vi "Simulador Circuito RLC-2.0.vi"() -> ()   [LabVIEW 2020]
uses:
  <vilib>/Utility/file.llb/Read Delimited Spreadsheet (DBL).vi
  <vilib>/measure/NI_MABase.lvlib
panel:
  in  "C":dbl
  in  "L":dbl
  in  "R":dbl
  in  "Gerar ondas\nde saída":bool
  out "Tensão no Capacitor":cluster{dbl[], "Y":dbl[]}[](graph)
  out "Corrente":cluster{dbl[], "Y":dbl[]}[](graph)
  in  "Arquivo texto da onda":path
  out "Onda de entrada":cluster{dbl[], "Y":dbl[]}(graph)
  in  "Duty Cicle":dbl
  in  "Informação da amostragem":T1={"Taxa de amostragem"=1000.0, "N° de amostras"=10000.0} {"N° de amostras" format="%#.6g"; "Taxa de amostragem" format="%#.6g"}
  in  "Gerar onda \nde Entrada":bool
  in  "Tipo de Onda":u16(ring) items=["Onda qualquer", "Senoidal", "Quadrada", ""]
  in  "Amplitude":dbl
  in  "Frequência":dbl
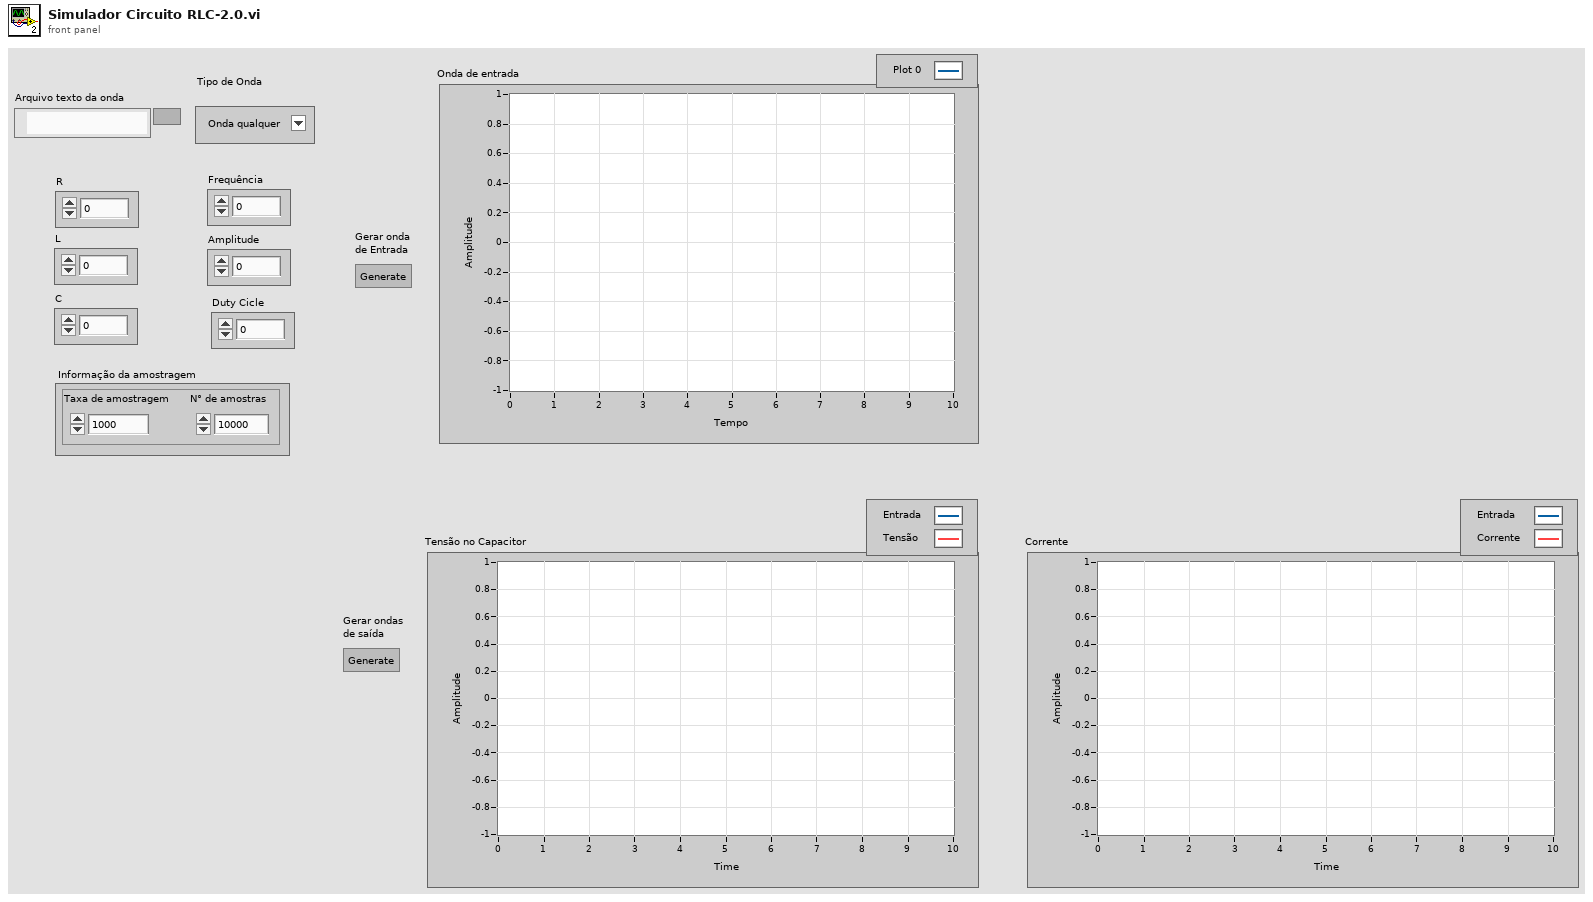
[diagram p1: front panel]
types:
  T1 = cluster{"Taxa de amostragem":dbl, "N° de amostras":dbl}
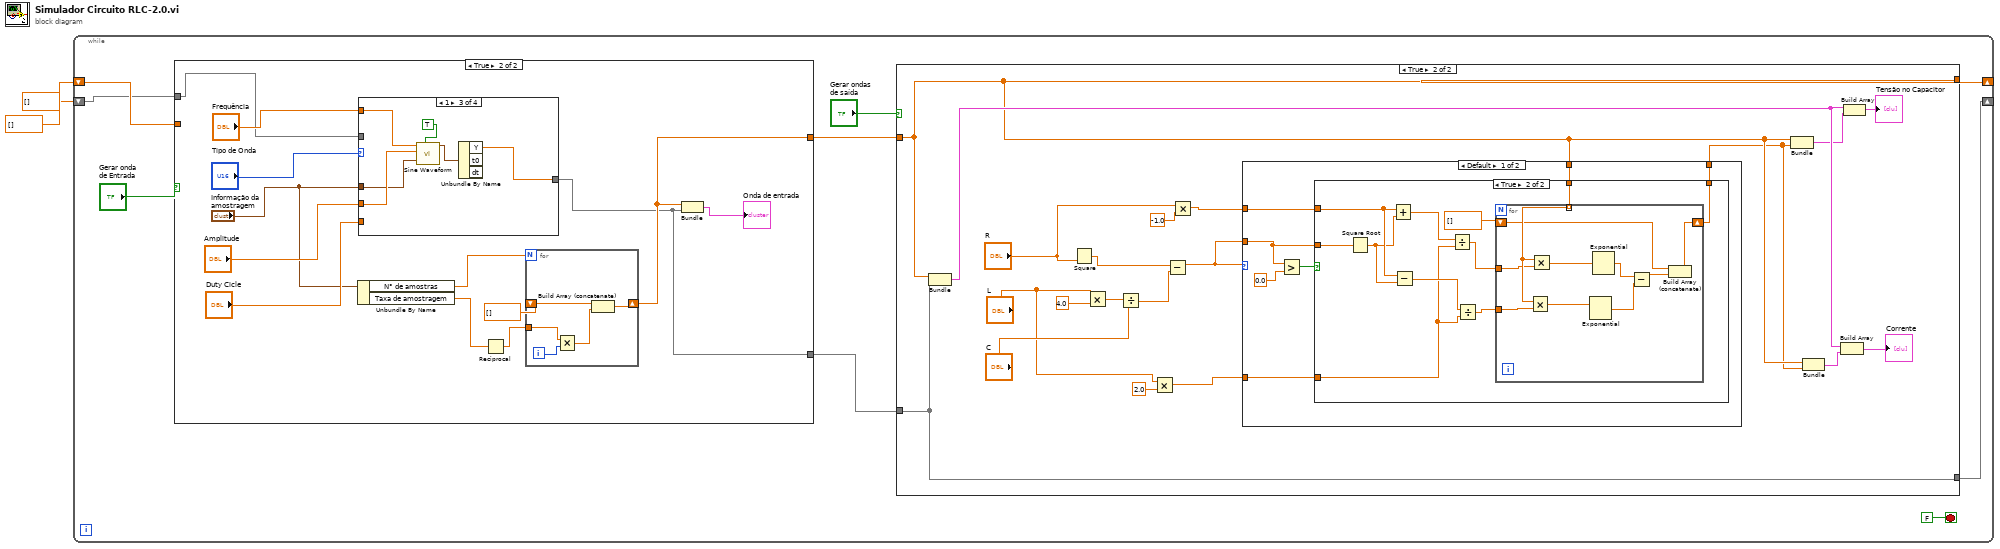
[diagram p0: block diagram]
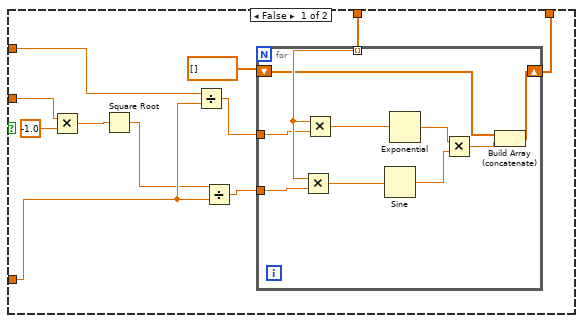
[diagram p3: hidden frame]
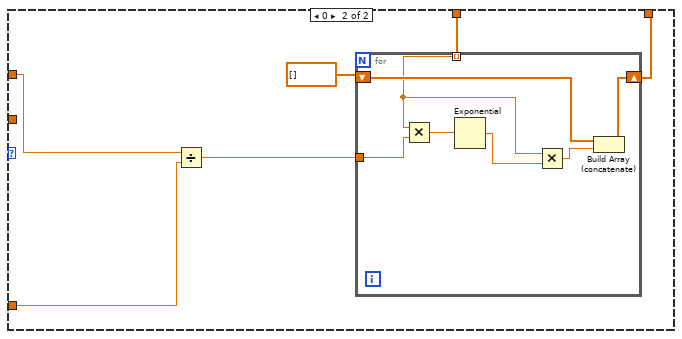
[diagram p4: hidden frame]
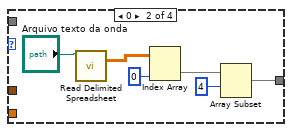
[diagram p7: hidden frame]
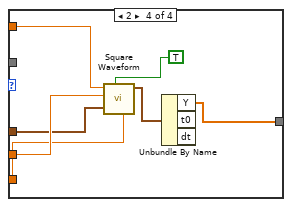
[diagram p8: hidden frame]
diagram:
  n1 = while {
    shift-right: [w6] -> _
    shift-left: dbl[] [] -> [w4]
    shift-right: [w5] -> _
    shift-left: dbl[] [] ("Y") -> [w3]
    stop <- FALSE stop-if-true
    n2 = case shown="True" "Gerar onda \nde Entrada" {
      tunnel: [w97 w100] -> w8
      tunnel: [w96 w99] -> w7
      tunnel: w4 -> [w97 _]
      tunnel: w3 -> [w96 w98]
      frame False {
      }
      frame True {
        n3 = Unbundle By Name("Informação da amostragem") -> ("N° de amostras"=w104:dbl, "Taxa de amostragem"=w105:dbl)
        n4 = case shown="1" "Tipo de Onda" {
          tunnel: "Amplitude" -> [_ _ w127 w134]
          tunnel: "Frequência" -> [_ _ w128 w135]
          tunnel: w98 -> [w116 _ _ _]
          tunnel: "Informação da amostragem" -> [_ _ w126 w133]
          tunnel: "Duty Cicle" -> [_ _ _ w132]
          tunnel: [w116 w117 w123 w129] -> w99
          frame Default {
          }
          frame 0 {
            n5 = call-poly <vilib>:"Read Delimited Spreadsheet.vi"("file path (dialog if empty)"="Arquivo texto da onda") -> ("all rows"=w121:dbl[][])  [unwired: 9 in, 5 out]
            n6 = Index Array(array=w121, index (col)=0 ("disabled index (col)")) -> (element=w118:dbl[])  [unwired: 1 in]
            n7 = Array Subset(array=w118, index=4) -> (w117:dbl[])  [unwired: 1 in]
          }
          frame 1 {
            n8 = call <vilib>:"Sine Waveform.vi"("sampling info"=w126, "reset signal"=TRUE, "amplitude"=w127, "frequency"=w128) -> ("signal out"=w124:waveform(dbl))  [unwired: 6 in, 1 out]
            n9 = Unbundle By Name(w124) -> ("Y"=w123:dbl[])  [unwired: 2 out]
          }
          frame 2 {
            n10 = call <vilib>:"Square Waveform.vi"("duty cycle (%)"=w132, "sampling info"=w133, "reset signal"=TRUE, "amplitude"=w134, "frequency"=w135) -> ("signal out"=w130:waveform(dbl))  [unwired: 5 in, 1 out]
            n11 = Unbundle By Name(w130) -> ("Y"=w129:dbl[])  [unwired: 2 out]
          }
        }
        n12 = Reciprocal(x=w105) -> (1/x=w103:dbl)
        n13 = for {
          N: w104 -> [_]
          tunnel: w103 -> [w114]
          shift-right: [w112] -> w100
          shift-left: dbl[] [] -> [w111]
          i -> [w115]
          n14 = Multiply(x=w114, y=w115) -> (x*y=w113:dbl)
          n15 = Build Array (concatenate)(w111, w113) -> (w112:dbl[])
        }
        n16 = Bundle(w100, "Y"=w99) -> (→"Onda de entrada":cluster{dbl[], "Y":dbl[]})  [unwired: 1 in]
      }
    }
    n17 = case shown="True" "Gerar ondas\nde saída" {
      tunnel: w8 -> [w13 w21]
      tunnel: w7 -> [w12 w31]
      tunnel: [w13 w21] -> w6
      tunnel: [w12 w31] -> w5
      frame False {
      }
      frame True {
        n18 = Bundle(w21, "Y"=w31) -> (w32:cluster{dbl[], "Y":dbl[]})  [unwired: 1 in]
        n19 = Square(x="R") -> (x^2=w27:dbl)
        n20 = Multiply(x="L", y=4.0) -> (x*y=w29:dbl)
        n21 = Divide(x=w29, y="C") -> (x/y=w26:dbl)
        n22 = Multiply(x="L", y=2.0) -> (x*y=w22:dbl)
        n23 = Subtract(x=w27, y=w26) -> (x-y=w14:dbl)
        n24 = Multiply(x="R", y=-1.0) -> (x*y=w23:dbl)
        n25 = case shown="Default" w14 {
          tunnel: w14 -> [w38 _]
          tunnel: w23 -> [w37 w88]
          tunnel: w22 -> [w36 w87]
          tunnel: w21 -> [w35 w84]
          tunnel: [w34 w83] -> w20
          frame Default {
            n26 = Greater?(x=w38, y=0.0) -> (0:w40:bool)
            n27 = case shown="True" w40 {
              tunnel: w38 -> [w44 w72]
              tunnel: w37 -> [w45 w71]
              tunnel: w36 -> [w47 w67]
              tunnel: w35 -> [w48 w66]
              tunnel: [w46 w62] -> w34
              frame False {
                n28 = Multiply(x=w44, y=-1.0) -> (x*y=w42:dbl)
                n29 = Square Root(x=w42) -> (sqrt(x)=w41:dbl)
                n30 = Divide(x=w45, y=w47) -> (x/y=w51:dbl)
                n31 = Divide(x=w41, y=w47) -> (x/y=w50:dbl)
                n32 = for {
                  tunnel: w48 -> [w61] mode=indexing
                  tunnel: w51 -> [w60]
                  tunnel: w50 -> [w59]
                  shift-right: [w52] -> w46
                  shift-left: dbl[] [] -> [w58]
                  n33 = Multiply(x=w61, y=w59) -> (x*y=w56:dbl)
                  n34 = Multiply(x=w61, y=w60) -> (x*y=w57:dbl)
                  n35 = Sine(x=w56) -> (sin(x)=w54:dbl)
                  n36 = Exponential(1:w57) -> (0:w55:dbl)
                  n37 = Multiply(x=w55, y=w54) -> (x*y=w53:dbl)
                  n38 = Build Array (concatenate)(w58, w53) -> (w52:dbl[])
                }
              }
              frame True {
                n39 = Square Root(x=w72) -> (sqrt(x)=w70:dbl)
                n40 = Add(x=w71, y=w70) -> (x+y=w69:dbl)
                n41 = Subtract(x=w71, y=w70) -> (x-y=w68:dbl)
                n42 = Divide(x=w69, y=w67) -> (x/y=w65:dbl)
                n43 = Divide(x=w68, y=w67) -> (x/y=w64:dbl)
                n44 = for {
                  tunnel: w66 -> [w82] mode=indexing
                  tunnel: w65 -> [w81]
                  tunnel: w64 -> [w80]
                  shift-right: [w78] -> w62
                  shift-left: dbl[] [] -> [w77]
                  n45 = Multiply(x=w82, y=w80) -> (x*y=w73:dbl)
                  n46 = Multiply(x=w82, y=w81) -> (x*y=w74:dbl)
                  n47 = Exponential(1:w73) -> (0:w75:dbl)
                  n48 = Exponential(1:w74) -> (0:w76:dbl)
                  n49 = Subtract(x=w76, y=w75) -> (x-y=w79:dbl)
                  n50 = Build Array (concatenate)(w77, w79) -> (w78:dbl[])
                }
              }
            }
          }
          frame 0 {
            n51 = Divide(x=w88, y=w87) -> (x/y=w85:dbl)
            n52 = for {
              shift-right: [w89] -> w83
              shift-left: dbl[] [] -> [w95]
              tunnel: w85 -> [w93]
              tunnel: w84 -> [w91] mode=indexing
              n53 = Multiply(x=w91, y=w93) -> (x*y=w94:dbl)
              n54 = Exponential(1:w94) -> (0:w92:dbl)
              n55 = Multiply(x=w91, y=w92) -> (x*y=w90:dbl)
              n56 = Build Array (concatenate)(w95, w90) -> (w89:dbl[])
            }
          }
        }
        n57 = Bundle(w21, w20) -> (w19:cluster{dbl[], dbl[]})  [unwired: 1 in]
        n58 = Bundle(w21, w20) -> (w18:cluster{dbl[], dbl[]})  [unwired: 1 in]
        n59 = Build Array(w32, w18) -> (→"Corrente":cluster{dbl[], "Y":dbl[]}[])
        n60 = Build Array(w32, w19) -> (→"Tensão no Capacitor":cluster{dbl[], "Y":dbl[]}[])
      }
    }
  }
